vi "Test Suite Error 7002 Message.vi"() -> ()   [LabVIEW 2013]
uses:
  classes/Test Suite/Test Suite.lvclass
panel:
  out "error out":errorcluster
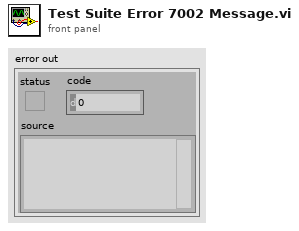
[diagram p1: front panel]
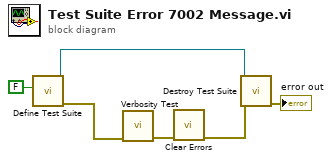
[diagram p0: block diagram]
diagram:
  n1 = call "Define Test Suite.vi"("Interactive"=FALSE) -> ("error out"=w6:errorcluster, "Test Suite"=w5:refnum<class "Test Suite.lvclass">)  [unwired: 9 in]
  n2 = call "Verbosity Test.vi"("error in (no error)"=w6) -> ("error out"=w2:errorcluster)  [unwired: 10 in]
  n3 = call <vilib>:"Clear Errors.vi"("error in (no error)"=w2) -> ("error out"=w1:errorcluster)  [unwired: 6 in]
  n4 = call-dynamic "Destroy Test Suite.vi"("error in (no error)"=w1, "Test Suite in"=w5) -> ("error out"=→"error out":errorcluster)  [unwired: 9 in]
